vi "Estop check.vi"(8 "error in (no error)":errorcluster, 11 "controller in":refnum<k24>) -> (0 "error out":errorcluster, 3 "controller out":refnum<k24>)   [LabVIEW 2021, in "A3200.lvclass"]
uses:
  A3200.lvclass
  C:/Program Files (x86)/Aerotech/A3200/LabVIEW/2010/Bin/Aerotech.A3200.dll
  Program Files (x86)/Aerotech/A3200/LabVIEW/2010/Bin/Aerotech.A3200.dll
  Drivers/Aerotech A3200/Aerotech.lvlib
panel:
  out "Instructions":string
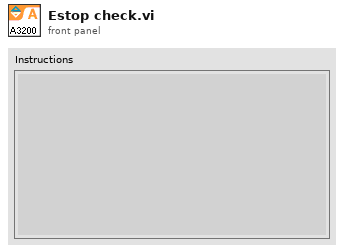
[diagram p1: front panel]
types:
  T1 = typedef "File Paths.ctl" = cluster{"Glue Pattern Folder":path, "Carrier Tray Folder":path, "Pick Up Tool Fixture Folder":path, "Components Folder":path, "Bellows Tool Offset.txt":path, "Pick Up Tool Offset.txt":path, "Dispense Tip Offset.txt":path, "Log Files":path, "Gantry Assembly Map.txt":path, "Syringe and offset map.txt":path, "Controllers Folder":path, "Local dbase config":path}
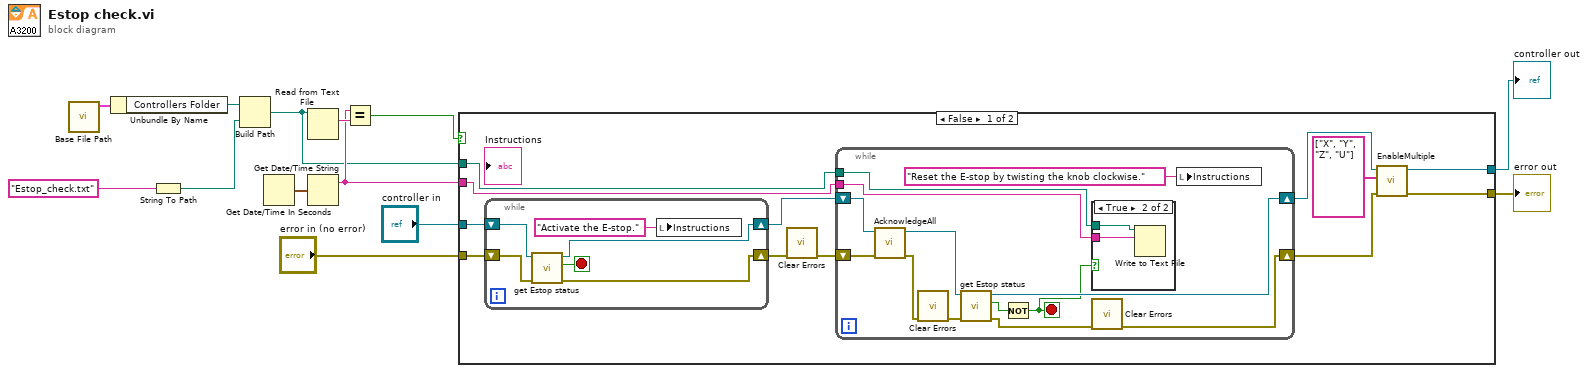
[diagram p0: block diagram]
diagram:
  n1 = call "Base File Path.vi"() -> ("Paths Out"=w9:T1)  [unwired: 11 in]
  n2 = Unbundle By Name(w9) -> ("Controllers Folder"=w8:path)
  n3 = String To Path(string="Estop_check.txt") -> (path=w7:path)
  n4 = Build Path(base path=w8, name or relative path=w7) -> (appended path=w1:path)
  n5 = Get Date/Time In Seconds() -> (seconds since 1Jan1904=w5:timestamp)
  n6 = Read from Text File(file (use dialog)=w1) -> (text=w4:string)  [unwired: 3 in, 3 out]
  n7 = Get Date/Time String(seconds (now)=w5) -> (date string=w2:string)  [unwired: 2 in, 1 out]
  n8 = Equal?(x=w2, y=w4) -> (x = y?=w3:bool)
  n9 = case shown="False" w3 {
    tunnel: "controller in" -> [w22 w48]
    tunnel: [w21 w48] -> w12
    tunnel: "error in (no error)" -> [w20 w47]
    tunnel: [w18 w47] -> w10
    tunnel: w2 -> [w15 _]
    tunnel: w1 -> [w14 _]
    frame False {
      n10 = while {
        shift-right: [w45] -> w25
        shift-left: w22 -> [w46]
        shift-right: [w41] -> w17
        shift-left: w20 -> [w42]
        stop <- w44 stop-if-true
        n11 = call "get Estop status.vi"("error in (no error)"=w42, "controller in"=w46) -> ("error out"=w41:errorcluster, "Estop?"=w44:bool, "controller out"=w45:refnum<k24>)  [unwired: 7 in]
        n12 = local write "Instructions"("Activate the E-stop." ("Instructions")) -> ()
      }
      n13 = call <vilib>:"Clear Errors.vi"("error in (no error)"=w17) -> ("error out"=w16:errorcluster)  [unwired: 5 in, 1 out]
      n14 = while {
        shift-right: [w35] -> w23
        shift-left: w25 -> [w37]
        shift-right: [w29] -> w19
        shift-left: w16 -> [w33]
        tunnel: w15 -> [w27]
        tunnel: w14 -> [w26]
        stop <- w28 stop-if-true
        n15 = call "AcknowledgeAll.vi"("error in (no error)"=w33, "controller in"=w37) -> ("error out"=w32:errorcluster, "controller out"=w36:refnum<k24>)  [unwired: 8 in]
        n16 = call <vilib>:"Clear Errors.vi"("error in (no error)"=w32) -> ("error out"=w31:errorcluster)  [unwired: 5 in, 1 out]
        n17 = call "get Estop status.vi"("error in (no error)"=w31, "controller in"=w36) -> ("error out"=w30:errorcluster, "Estop?"=w38:bool, "controller out"=w35:refnum<k24>)  [unwired: 7 in]
        n18 = Not(x=w38) -> (.not. x?=w28:bool)
        n19 = case shown="True" w28 {
          tunnel: w27 -> [_ w40]
          tunnel: w26 -> [_ w39]
          frame False {
          }
          frame True {
            n20 = Write to Text File(file (use dialog)=w39, text=w40) -> ()  [unwired: 2 in, 3 out]
          }
        }
        n21 = call <vilib>:"Clear Errors.vi"("error in (no error)"=w30) -> ("error out"=w29:errorcluster)  [unwired: 5 in, 1 out]
        n22 = local write "Instructions"("Reset the E-stop by twisting the knob clockwise." ("Instructions")) -> ()
      }
      n23 = call "EnableMultiple.vi"("error in (no error)"=w19, "axis names"=string[] ["X", "Y", "Z", "U"], "controller in"=w23) -> ("error out"=w18:errorcluster, "controller out"=w21:refnum<k24>)  [unwired: 7 in]
    }
    frame True {
    }
  }
  "controller out" <- w12
  "error out" <- w10
